vi "Read Multi Time.vi"(8 "error in (no error)":errorcluster, 9 "Type":timestamp[](array[timestamp]), 10 "Tag":string[](array[string]), 11 "Var Bus in":refnum<class "Omni_Bus.lvclass">) -> (0 "error out":errorcluster, 2 "Times":timestamp[](array[timestamp]), 3 "Var Bus out":refnum<class "Omni_Bus.lvclass">)   [LabVIEW 2021, in "Omni_Bus.lvclass"]
uses:
  Omni_Bus.lvclass
  <vilib>/TSA/Abstract Data Classes/Abs_Types/Time/Abs_Time.lvclass
  C:/Program Files (x86)/National Instruments/LabVIEW 2021/vi.lib/TSA/Abstract Data Classes/Abs_Types/Type/Abs_Type.lvclass
  <vilib>/TSA/Abstract Data Classes/Abs_Types/Type/Abs_Type.lvclass/Abs_Type.ctl
  Omni_Bus.lvclass/Omni_Bus.ctl
  FindMultiVar.vi
  FindVar.vi
  <vilib>/Utility/error.llb/Clear Errors.vi
  Properties/Read Var Map.vi
  <vilib>/TSA/Abstract Data Classes/Abs_Types/Type/Properties/Read Tag.vi
  <vilib>/TSA/Abstract Data Classes/Abs_Types/Value/Abs_Value.lvclass
  Check For Read Only Error.vi
  Incorrect Tag String Error.vi
  <vilib>/TSA/Abstract Data Classes/Abs_Types/Type/Abs_Type.lvclass
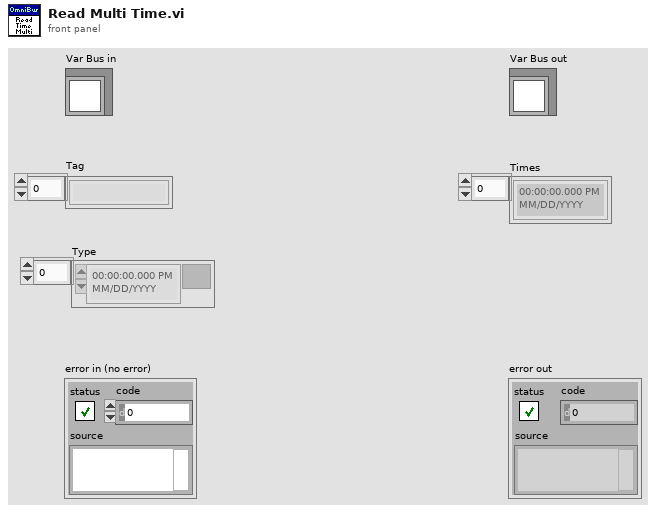
[diagram p1: front panel]
types:
  T1 = typedef "Abs_Time.lvclass/Type.ctl" = timestamp
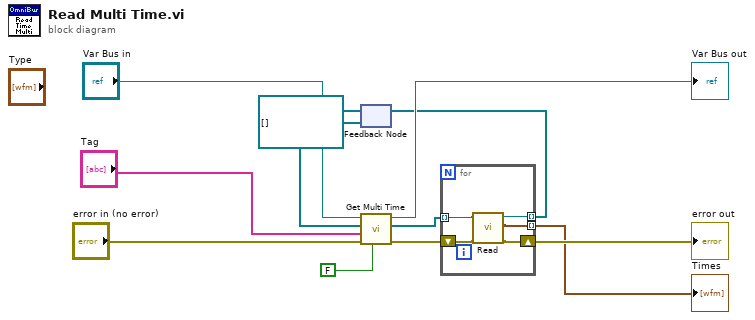
[diagram p0: block diagram]
diagram:
  n1 = feedback #1(refnum<class "Abs_Time.lvclass">[] []) -> (w8:refnum<class "Abs_Time.lvclass">[])
  n2 = call "Get Multi Time.vi"("Write?"=FALSE, "error in (no error)"="error in (no error)", "Tag"="Tag", "Value Type"=w8, "Var Bus in"="Var Bus in") -> ("error out"=w7:errorcluster, "Value Out"=w6:refnum<class "Abs_Time.lvclass">[], "Var Bus out"=→"Var Bus out":refnum<class "Omni_Bus.lvclass">)  [unwired: 3 in, 1 out]
  n3 = for {
    tunnel: w6 -> [w16] mode=indexing
    tunnel: [w14] -> w4 mode=indexing
    tunnel: [w13] -> w3 mode=indexing
    shift-right: [w15] -> w5
    shift-left: w7 -> [w17]
    n4 = call-dynamic "Read.vi"("error in (no error)"=w17, "Double Float.lvclass_340760 in"=w16) -> ("error out"=w15:errorcluster, "Value"=w13:T1, "Double Float.lvclass_340760 out"=w14:refnum<class "Abs_Time.lvclass">)  [unwired: 7 in]
  }
  "error out" <- w5
  "Times" <- w3
  n5 = feedback-in #1(w4) -> ()
